vi "Pressure.vi"(8 "error in (no error)":errorcluster, 10 "Pressure":i16, 11 "Ultimus V in":refnum<class "Ultimus V2.lvclass">) -> (0 "error out":errorcluster, 3 "Ultimus V out":refnum<class "Ultimus V2.lvclass">)   [LabVIEW 2016, in "Ultimus V2.lvclass"]
uses:
  Ultimus V2.lvclass
  Ultimus V2.lvclass/Ultimus V2.ctl
  Drivers/EFD Ultimus V/EFD Ultimus V.lvlib
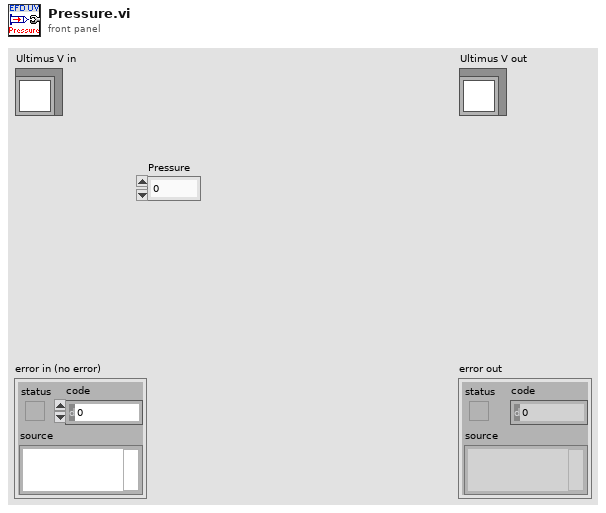
[diagram p1: front panel]
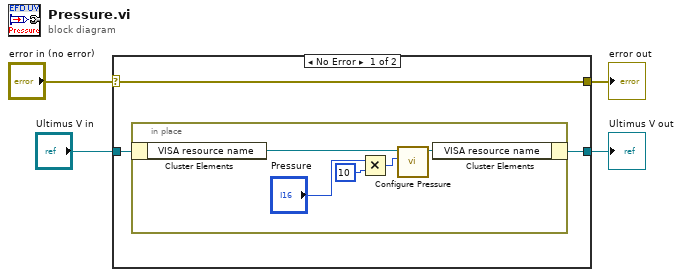
[diagram p0: block diagram]
diagram:
  n1 = case shown="No Error" "error in (no error)" {
    selector: "error in (no error)" -> [w5 w14]
    tunnel: "Ultimus V in" -> [w7 w13]
    tunnel: [w6 w13] -> w3
    tunnel: [w5 w14] -> w1
    frame No Error {
      n2 = in-place {
        n3 = in-place-cluster #1(w7) -> ("VISA resource name"=w12:refnum<visa-resource-name>)
        n4 = Multiply(x="Pressure", y=i16 10) -> (x*y=w8:i16)
        n5 = call "Configure Pressure.vi"("Pressure Setting (0000)"=w8, "VISA resource name"=w12) -> ("VISA resource name out"=w11:refnum<visa-resource-name>)  [unwired: 8 in, 1 out]
        n6 = in-place-cluster #1("VISA resource name"=w11) -> (w6:refnum<class "Ultimus V2.lvclass">)
      }
    }
    frame Error {
    }
  }
  "error out" <- w1
  "Ultimus V out" <- w3
